vi "draw_circle_on_section.vi"(8 "Error In":errorcluster, 10 "Parameters":T1, 11 "Image Src":T2) -> (0 "Error Out":errorcluster, 3 "Image Dst Out":T2)   [LabVIEW 2019]
uses:
  <vilib>/vision/Image Controls.llb/IMAQ Image.ctl
  parameters_cluster_typedef.ctl
  <vilib>/vision/NI_Vision_Development_Module.lvlib
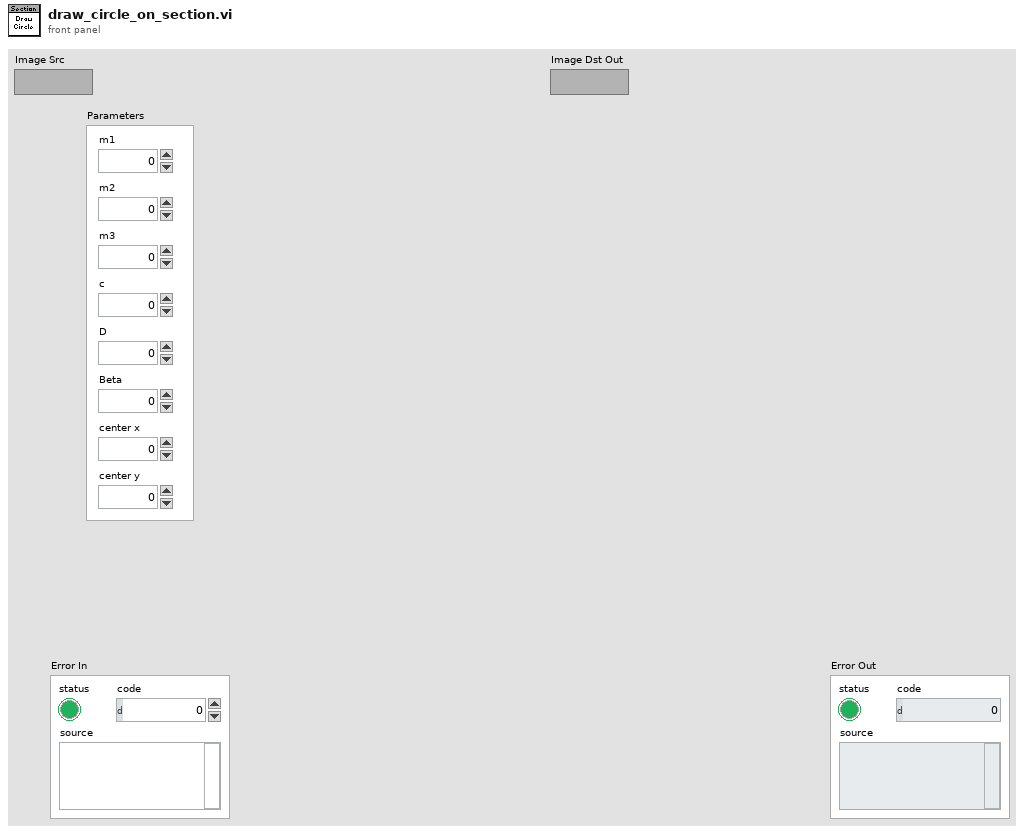
[diagram p1: front panel]
types:
  T1 = typedef "parameters_cluster_typedef.ctl" = cluster{"m1":dbl, "m2":dbl, "m3":dbl, "c":dbl, "D":dbl, "Beta":dbl, "center x":dbl, "center y":dbl}
  T2 = typedef "IMAQ Image.ctl" = refnum<image>
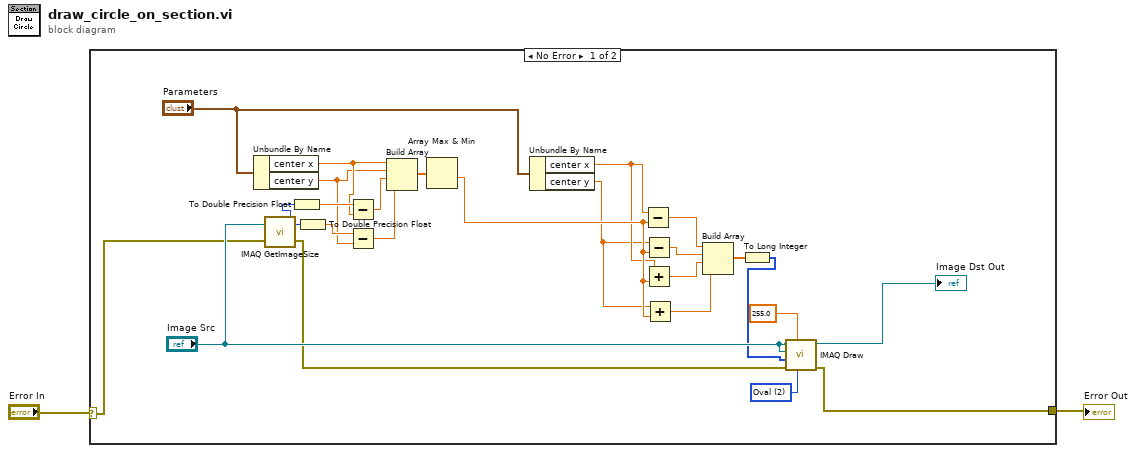
[diagram p0: block diagram]
diagram:
  n1 = case shown="No Error" "Error In" {
    selector: "Error In" -> [w4 w28]
    tunnel: [w3 w28] -> w1
    frame No Error {
      w27 = u16 2 items=["Line", "Rectangle", "Oval"] ("Shape to draw")
      n2 = Unbundle By Name("Parameters") -> ("center x"=w21:dbl, "center y"=w19:dbl)
      n3 = call "IMAQ GetImageSize"("Image"="Image Src", "error in (no error)"=w4) -> ("Y Resolution"=w23:i32, "error out"=w8:errorcluster)  [unwired: 2 in, 1 out]
      n4 = To Double Precision Float(number=w23) -> (double precision float=w22:dbl)
      n5 = To Double Precision Float(number=w23) -> (double precision float=w20:dbl)
      n6 = Subtract(x=w22, y=w21) -> (x-y=w25:dbl)
      n7 = Subtract(x=w20, y=w19) -> (x-y=w24:dbl)
      n8 = Build Array(w21, w19, w25, w24) -> (w18:dbl[])
      n9 = Array Max & Min(array=w18) -> (min value=w16:dbl)  [unwired: 3 out]
      n10 = Unbundle By Name("Parameters") -> ("center x"=w15:dbl, "center y"=w14:dbl)
      n11 = Subtract(x=w15, y=w16) -> (x-y=w13:dbl)
      n12 = Subtract(x=w14, y=w16) -> (x-y=w12:dbl)
      n13 = Add(x=w15, y=w16) -> (x+y=w11:dbl)
      n14 = Add(x=w14, y=w16) -> (x+y=w10:dbl)
      n15 = Build Array(w13, w12, w11, w10) -> (w6:dbl[])
      n16 = To Long Integer(number=w6) -> (32bit integer=w5:i32[])
      n17 = call "IMAQ Draw"("Shape to draw"=w27, "Pixel Color"=sgl 255.0, "error in (no error)"=w8, "Coordinates"=w5, "Image Dst"="Image Src", "Image Src"="Image Src") -> ("error out"=w3:errorcluster, "Image Dst Out"=→"Image Dst Out":T2)  [unwired: 4 in]
    }
    frame Error {
    }
  }
  "Error Out" <- w1
